vi "Global_STOP.vi"() -> ()   [LabVIEW 2023]
panel:
  in  "STOP":bool
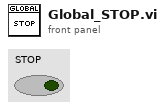
[diagram p1: front panel]
diagram:
